vi "FTW-Benchmark-MessageTransports.vi"() -> ()   [LabVIEW 2012]
uses:
  Actor/Utility/FTW-Actor-Address.ctl
  Actor/Utility/FTW-Actor-Configuration.ctl
  Actor/Endpoint/FTW-Endpoint.lvclass
  Actor/Message/Request/FTW-Message-IncomingRequest.lvclass
  Actor/FTW-Actor.lvlib
  Actor/Ether/FTW-Ether.lvclass
panel:
  in  "Client Mode":enum32{"Parallel", "Serial"}(radio)=enum."Serial"
  in  "Number of Clients":i32=8
  out "Results":T2(array[cluster])
  in  "Server Addresses to Test":T1[](array[typedef])=["tcp://127.0.0.1:*", "inproc://just-a-test", "lvq://just-a-named-queue"]
  in  "Requests to Send":i32=500
  in  "stop":bool
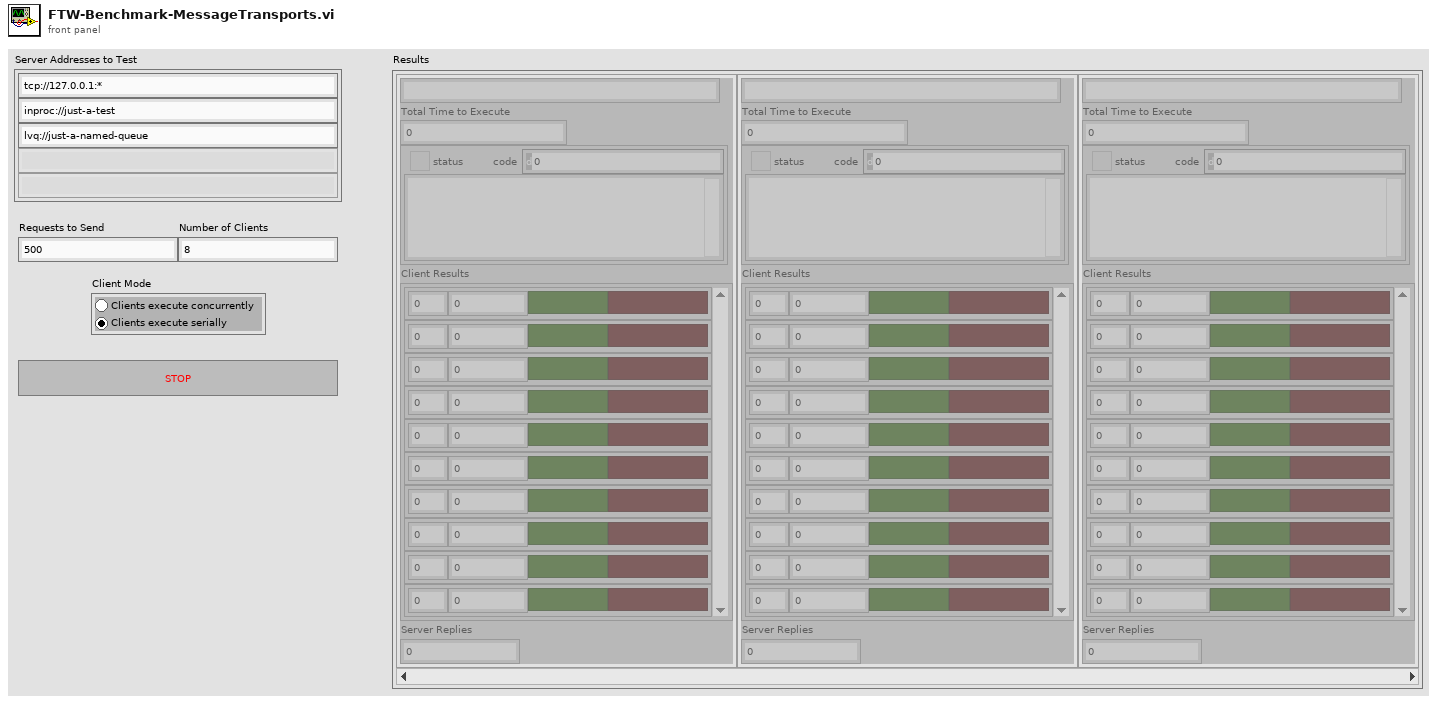
[diagram p1: front panel]
types:
  T1 = typedef "FTW-Actor.lvlib/FTW-Actor-Address.ctl" = string
  T2 = cluster{"Server Address":T1, "Total Time to Execute":u32, "error":errorcluster, "Client Results":cluster{"Instance":i32, "Requests":i32, "All replies were as expected?":bool, "Timed out?":bool}[], "Server Replies":i32}[]
  T3 = typedef "FTW-Actor.lvlib/FTW-Actor-Configuration.ctl" = string
  T4 = cluster{"Actual Endpoint Address":T1, "Elapsed Time":u32, "error out":errorcluster, cluster{i32, i32, bool, bool}[], i32}[]
  T5 = cluster{"Actual Server Address":T1, "Elapsed Time":u32, "error IO":errorcluster, cluster{i32, i32, bool, bool}[], i32}
  T6 = cluster{"Actual Server Address":T1, "Elapsed Time":u32, "error IO":errorcluster, cluster{i32, i32, bool, bool}[], i32}[]
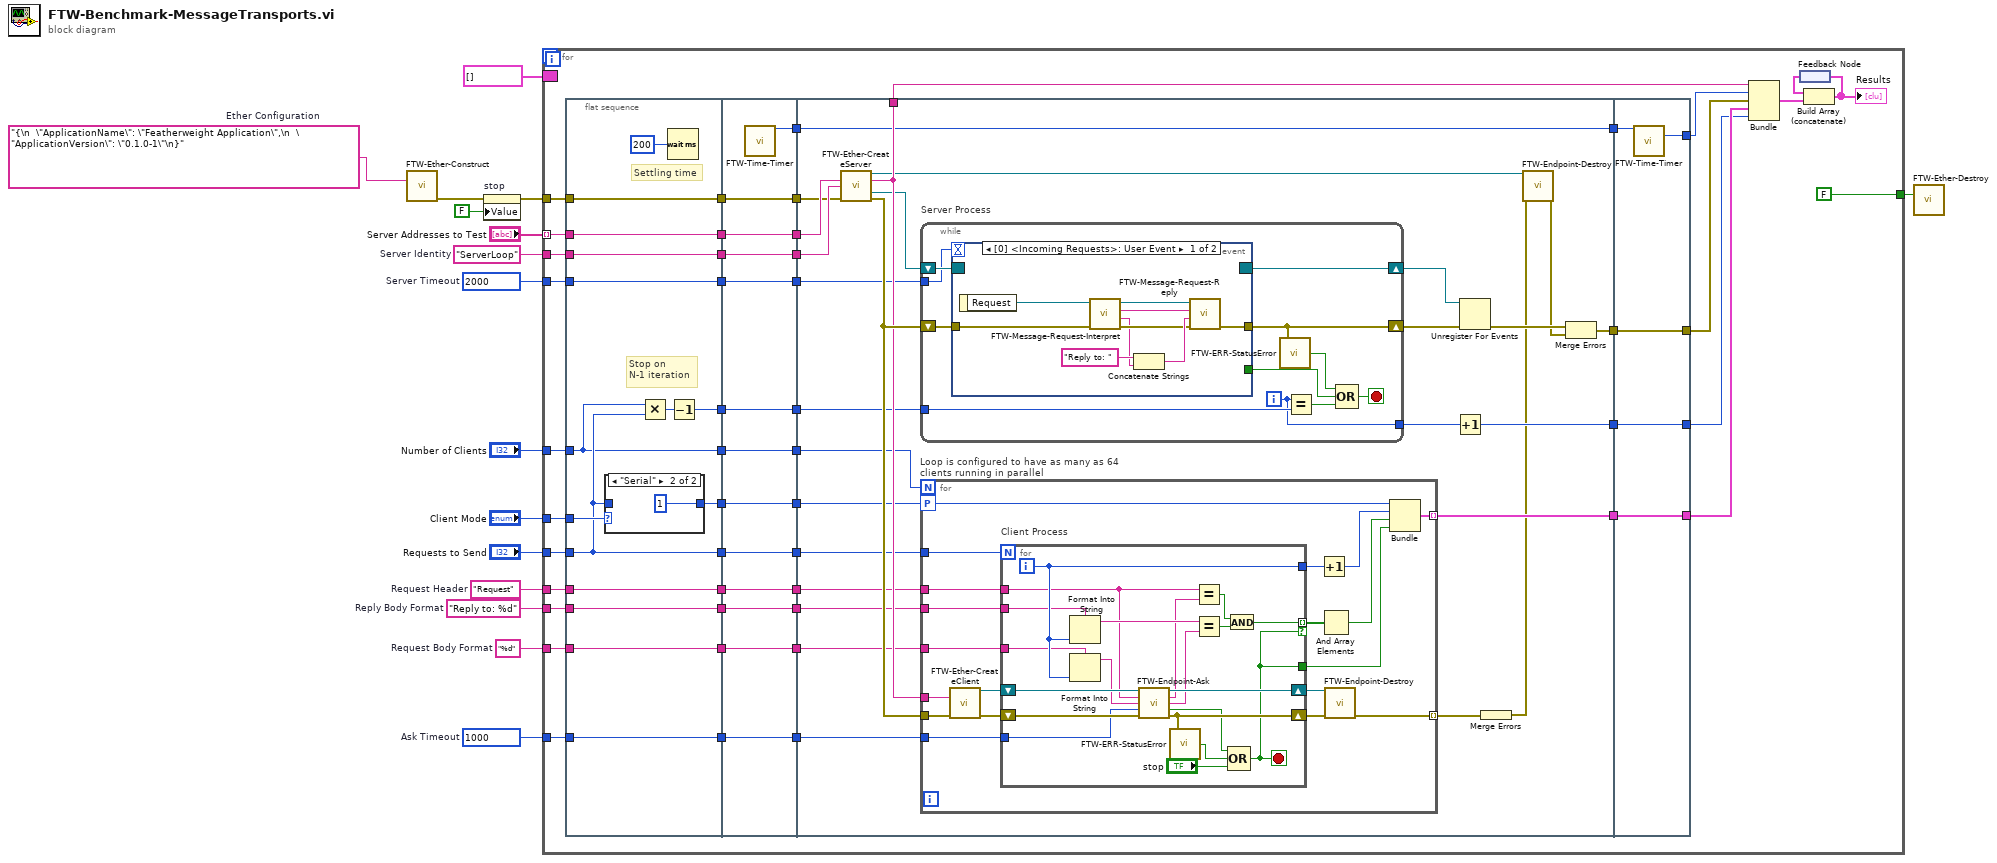
[diagram p0: block diagram]
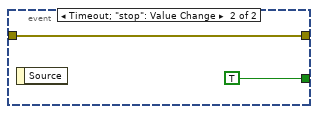
[diagram p3: hidden frame]
diagram:
  w1 = T3 "{\n  \"ApplicationName\": \"Featherweight Application\",\n  \"ApplicationVersion\": \"0.1.0-1\"\n}"  # Ether Configuration
  w3 = "%d"  # Request Body Format
  w5 = "Request"  # Request Header
  w4 = "Reply to: %d"  # Reply Body Format
  w8 = 1000  # Ask Timeout
  w9 = 2000  # Server Timeout
  w13 = "ServerLoop"  # Server Identity
  n1 = call "FTW-Ether-Construct.vi"("Ether Configuration"=w1) -> ("error out"=w6:errorcluster)  [unwired: 14 in]
  n2 = property on="stop" class="Bool (strict)"(error in=w6, "Value"=FALSE ("stop")) -> (error out=w10:errorcluster)  [unwired: 1 in, 1 out]
  n3 = for {
    tunnel: "Server Addresses to Test" -> [w58] mode=indexing
    tunnel: "Number of Clients" -> [w53]
    tunnel: "Requests to Send" -> [w46]
    tunnel: w13 -> [w42]
    tunnel: "Client Mode" -> [w41]
    tunnel: w10 -> [w40]
    tunnel: w9 -> [w37]
    tunnel: w8 -> [w34]
    border: T4 [] -> [_]
    tunnel: w5 -> [w24]
    tunnel: w4 -> [w21]
    tunnel: w3 -> [w18]
    tunnel: [FALSE ("Force Destroy?")] -> w2
    n4 = flat-sequence {
      tunnel: [w80] -> w65
      tunnel: [w78] -> w59
      tunnel: [w66] -> w54
      tunnel: [w70] -> w47
      tunnel: [w77] -> w43
      tunnel: w40 -> [w80]
      tunnel: w41 -> [w74]
      tunnel: w42 -> [w77]
      tunnel: w46 -> [w70]
      tunnel: w53 -> [w66]
      tunnel: w58 -> [w78]
      tunnel: [w76] -> w38
      tunnel: w37 -> [w76]
      tunnel: [w75] -> w35
      tunnel: w34 -> [w75]
      tunnel: [w73] -> w32
      tunnel: [w71] -> w30
      tunnel: [w69] -> w25
      tunnel: w24 -> [w69]
      tunnel: [w68] -> w22
      tunnel: w21 -> [w68]
      tunnel: [w67] -> w19
      tunnel: w18 -> [w67]
      tunnel: [w95] -> w64
      tunnel: [w94] -> w63
      tunnel: w65 -> [w95]
      tunnel: [w93] -> w60
      tunnel: w59 -> [w93]
      tunnel: [w92] -> w55
      tunnel: w54 -> [w92]
      tunnel: [w91] -> w48
      tunnel: w47 -> [w91]
      tunnel: [w90] -> w44
      tunnel: w43 -> [w90]
      tunnel: [w89] -> w39
      tunnel: w38 -> [w89]
      tunnel: [w88] -> w36
      tunnel: w35 -> [w88]
      tunnel: [w87] -> w33
      tunnel: w32 -> [w87]
      tunnel: [w86] -> w31
      tunnel: w30 -> [w86]
      tunnel: [w85] -> w26
      tunnel: w25 -> [w85]
      tunnel: [w84] -> w23
      tunnel: w22 -> [w84]
      tunnel: [w83] -> w20
      tunnel: w19 -> [w83]
      tunnel: [w99] -> w62
      tunnel: [w118] -> w61
      tunnel: [w117] -> w51
      tunnel: [w116] -> w50
      tunnel: w31 -> [w112]
      tunnel: w33 -> [w103]
      tunnel: w64 -> [w100]
      tunnel: w63 -> [w118]
      tunnel: w60 -> [w102]
      tunnel: w55 -> [w109]
      tunnel: w48 -> [w111]
      tunnel: [w121] -> w45
      tunnel: w44 -> [w101]
      tunnel: w39 -> [w108]
      tunnel: w36 -> [w107]
      tunnel: w26 -> [w98]
      tunnel: w23 -> [w97]
      tunnel: w20 -> [w96]
      tunnel: [w188] -> w57
      tunnel: w62 -> [w188]
      tunnel: w61 -> [w187]
      tunnel: [w186] -> w56
      tunnel: [w185] -> w52
      tunnel: w51 -> [w185]
      tunnel: [w184] -> w49
      tunnel: w50 -> [w184]
      frame #0 {
        # "Stop on\nN-1 iteration"
        # "Settling time"
        n5 = case shown="\"Serial\"" w74 {
          tunnel: w70 -> [w81 _]
          tunnel: [w81 1 ("Requests to Send")] -> w73
          frame "Parallel" {
          }
          frame "Serial" {
          }
        }
        n6 = Multiply(x=w66, y=w70) -> (x*y=w72:i32)
        n7 = Wait (ms)(milliseconds to wait=u32 200) -> ()  [unwired: 1 out]
        n8 = Decrement(x=w72) -> (x-1=w71:i32)
      }
      frame #1 {
        n9 = call "FTW-Time-Timer.vi"() -> ("Current Tick Count"=w94:u32)  [unwired: 13 in, 2 out]
      }
      frame #2 {
        n10 = call "FTW-Ether-CreateServer.vi"("Server Address"=w102, "Server Identity"=w101, "error in"=w100) -> ("Server Endpoint"=w106:refnum<class "FTW-Endpoint.lvclass">, "Actual Server Address"=w121:T1, "Incoming Requests"=w113:refnum<event-registration>, "error out"=w122:errorcluster)  [unwired: 8 in, 1 out]
        n11 = while "Server Process" {
          shift-right: [w171] -> w114
          shift-left: w113 -> [w172]
          shift-right: [w169] -> w115
          shift-left: w122 -> [w170]
          tunnel: w112 -> [w164]
          tunnel: [w163] -> w110
          tunnel: w108 -> [w162]
          i -> [w163]
          stop <- w165 stop-if-true
          n12 = event shown="[0] <Incoming Requests>: User Event" {
            selector: w172 -> [_ _]
            dyn-events: [_ _] -> w171
            timeout: w162 -> [_ _]
            tunnel: [_ TRUE] -> w167
            tunnel: w170 -> [w177 w182]
            tunnel: [w179 w182] -> w169
            event User Event {
              n13 = event-data() -> ("Request"=w180:refnum<class "FTW-Message-IncomingRequest.lvclass">)  [unwired: 1 in]
              n14 = call "FTW-Message-Request-Interpret.vi"("error in"=w177, "FTW Incoming Request"=w180) -> ("error out"=w176:errorcluster, "Request Body"=w173:string, "Request Header"=w174:string, "FTW Request"=w175:refnum<class "FTW-Message-IncomingRequest.lvclass">)  [unwired: 6 in]
              n15 = Concatenate Strings("Reply to: ", w173) -> (w178:string)
              n16 = call "FTW-Message-Request-Reply.vi"("error in"=w176, "Response Body"=w178, "Response Header"=w174, "FTW Incoming Request"=w175) -> ("error out"=w179:errorcluster)  [unwired: 6 in, 1 out]
            }
            event Timeout; "stop": Value Change {
              n17 = event-data() -> ()  [unwired: 1 in, 1 out]
            }
          }
          n18 = call "FTW-ERR-StatusError.vi"("error to check"=w169) -> ("Error?"=w168:bool)
          n19 = Equal?(x=w163, y=w164) -> (x = y?=w166:bool)
          n20 = Compound Arithmetic op=OR(w168, w167, w166) -> (w165:bool)
        }
        n21 = for "Loop is configured to have as many as 64 clients running in parallel" {
          N: w109 -> [_]
          tunnel: w122 -> [w125]
          tunnel: w111 -> [w141]
          tunnel: w107 -> [w140]
          workers-P: w103 -> [w134]
          tunnel: [w138] -> w105 mode=indexing
          tunnel: [w137] -> w117 mode=indexing
          tunnel: w121 -> [w123]
          tunnel: w97 -> [w132]
          tunnel: w98 -> [w131]
          tunnel: w96 -> [w130]
          n22 = call "FTW-Ether-CreateClient.vi"("Server Address"=w123, "error in"=w125) -> ("Client Endpoint"=w126:refnum<class "FTW-Endpoint.lvclass">, "error out"=w124:errorcluster)  [unwired: 12 in]
          n23 = for "Client Process" {
            N: w141 -> [_]
            shift-right: [w159] -> w139
            shift-left: w126 -> [w161]
            tunnel: w140 -> [w155]
            tunnel: [w150] -> w135
            tunnel: [w153] -> w136
            tunnel: [w146] -> w129 mode=indexing if=w150
            tunnel: w132 -> [w152]
            tunnel: w131 -> [w142]
            tunnel: w130 -> [w151]
            shift-right: [w158] -> w127
            shift-left: w124 -> [w160]
            i -> [w153]
            stop <- w150 stop-if-true
            n24 = Format Into String(format string=w152, w153) -> (resulting string=w145:string)  [unwired: 2 in, 1 out]
            n25 = Format Into String(format string=w151, w153) -> (resulting string=w149:string)  [unwired: 2 in, 1 out]
            n26 = call-dynamic "FTW-Endpoint-Ask.vi"("FTW Endpoint"=w161, "Request Header"=w142, "Request Body"=w149, "Timeout"=w155, "error in"=w160) -> ("FTW Endpoint out"=w159:refnum<class "FTW-Endpoint.lvclass">, "Response Header"=w144:string, "Response Body"=w143:string, "Timed out?"=w154:bool, "error out"=w158:errorcluster)  [unwired: 6 in]
            n27 = call "FTW-ERR-StatusError.vi"("error to check"=w158) -> ("Error?"=w157:bool)
            n28 = Equal?(x=w142, y=w144) -> (x = y?=w147:bool)
            n29 = Equal?(x=w145, y=w143) -> (x = y?=w148:bool)
            n30 = And(x=w147, y=w148) -> (x .and. y?=w146:bool)
            n31 = Compound Arithmetic op=OR(w154, w157, "stop") -> (w150:bool)
          }
          n32 = Increment(x=w136) -> (x+1=w133:i32)
          n33 = And Array Elements(Boolean array=w129) -> (logical AND=w128:bool)
          n34 = call-dynamic "FTW-Endpoint-Destroy.vi"("FTW Endpoint Type"=w139, "error in"=w127) -> ("error out"=w138:errorcluster)  [unwired: 13 in]
          n35 = Bundle(w134, w133, w128, w135) -> (w137:cluster{i32, i32, bool, bool})  [unwired: 1 in]
        }
        n36 = Increment(x=w110) -> (x+1=w116:i32)
        n37 = Unregister For Events(event registration refnum=w114, error in=w115) -> (error out=w120:errorcluster)
        n38 = Merge Errors(w105) -> (w104:errorcluster)
        n39 = call-dynamic "FTW-Endpoint-Destroy.vi"("FTW Endpoint Type"=w106, "error in"=w104) -> ("error out"=w119:errorcluster)  [unwired: 13 in]
        n40 = Merge Errors(w120, w119) -> (w99:errorcluster)
      }
      frame #3 {
        n41 = call "FTW-Time-Timer.vi"("Initial Tick Count"=w187) -> ("Elapsed Time"=w186:u32)  [unwired: 12 in, 2 out]
      }
    }
    n42 = Bundle("Actual Server Address"=w45, "Elapsed Time"=w56, "error IO"=w57, w52, w49) -> (w29:T5)  [unwired: 1 in]
    n43 = feedback #1() -> (w28:T4)
    n44 = Build Array (concatenate)(w28, w29) -> (w27:T6)
    "Results" <- w27
    n45 = feedback-in #1(w27) -> ()
  }
  n46 = call "FTW-Ether-Destroy.vi"("Force Destroy?"=w2) -> ()  [unwired: 14 in, 1 out]
